vi "check _input.vi"(7 "max_d (m)":dbl=10.0 format="%#_13g", 10 "input":T1(array[cluster])=[{"final vel. (m/s)"=0.0, "distance (m)"=0.15, "hold (s)"=0.0}, {"final vel. (m/s)"=1000.0, "distance (m)"=0.05, "hold (s)"=0.0}]) -> (2 "valid":bool=TRUE)   [LabVIEW 2017, in "wf.lvlib" / "wf_tools.lvlib"]
uses:
  wf_tools.lvlib
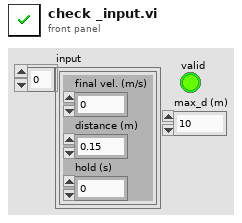
[diagram p1: front panel]
types:
  T1 = cluster{"final vel. (m/s)":dbl, "distance (m)":dbl, "hold (s)":dbl}[]
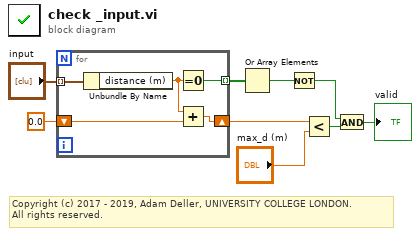
[diagram p0: block diagram]
diagram:
  # "Copyright (c) 2017 - 2019, Adam Deller, UNIVERSITY COLLEGE LONDON.\nAll rights reserved."
  n1 = for {
    tunnel: "input" -> [w14] mode=indexing
    tunnel: [w13] -> w8 mode=indexing
    shift-right: [w10] -> w5
    shift-left: 0.0 ("distance (m)") -> [w12]
    n2 = Unbundle By Name(w14) -> ("distance (m)"=w11:dbl)
    n3 = Equal To 0?(x=w11) -> (x = 0?=w13:bool)
    n4 = Add(x=w11, y=w12) -> (x+y=w10:dbl)
  }
  n5 = Or Array Elements(Boolean array=w8) -> (logical OR=w7:bool)
  n6 = Not(x=w7) -> (.not. x?=w2:bool)
  n7 = Less?(x=w5, y="max_d (m)") -> (x < y?=w3:bool)
  n8 = And(x=w2, y=w3) -> (x .and. y?=→"valid":bool)
